vi "SetValue.vi"(8 "error in":errorcluster, 10 "Value":T1=enum."NOT_COMPLETED", 11 "ExecutionStatus in":refnum<class "ExecutionStatus.lvclass">) -> (0 "error out":errorcluster, 3 "ExecutionStatus out":refnum<class "ExecutionStatus.lvclass">)   [LabVIEW 2021, in "ProligentXMLGenerator.lvlib" / "ExecutionStatus.lvclass"]
uses:
  ExecutionStatus.lvclass
  ExecutionStatus.lvclass/ExecutionStatus.ctl
  Value.ctl
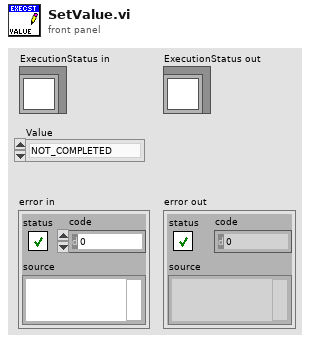
[diagram p1: front panel]
types:
  T1 = typedef "ProligentXMLGenerator.lvlib/ExecutionStatus.lvclass/Value.ctl" = enum16{"PASS", "FAIL", "NOT_COMPLETED", "ABORTED"}
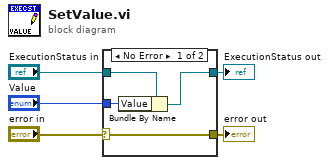
[diagram p0: block diagram]
diagram:
  n1 = case shown="No Error" "error in" {
    selector: "error in" -> [w6 w10]
    tunnel: "ExecutionStatus in" -> [w9 w11]
    tunnel: [w8 w11] -> w2
    tunnel: "Value" -> [w7 _]
    tunnel: [w6 w10] -> w1
    frame No Error {
      n2 = Bundle By Name(cluster=w9, "Value"=w7) -> (w8:refnum<class "ExecutionStatus.lvclass">)
    }
    frame Error {
    }
  }
  "error out" <- w1
  "ExecutionStatus out" <- w2
